vi "PathPlanner_PathFinder_GetGridPos.vi"(11 "RealGridPos":T2 {"Y" format="%14.3f"; "X" format="%14.3f"}) -> (1 "HashCode":i32, 3 "GridPosition":T1)   [LabVIEW 2019, in "PathPlanner24.lvlib"]
doc: "Internal function. Not to be used by end users."
uses:
  PathPlanner24.lvlib
  <vilib>/Rock Robotics/WPI/ThirdParty/JAS_Junk/TrajLib/TypeDef/TRANSLATION2D.ctl
  TypeDef/PathPlannerFinderGridPosition.ctl
  PathPlanner_GridPosition_Get.vi
  PathPlanner_PathFinder_Globals.vi
  <vilib>/Rock Robotics/WPI/ThirdParty/JAS_Junk/TrajLib/Trajectory_Library.lvlib
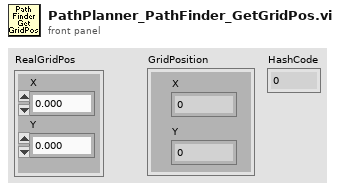
[diagram p1: front panel]
types:
  T1 = typedef "PathPlanner24.lvlib/PathPlannerFinderGridPosition.ctl" = cluster{"X":i32, "Y":i32}
  T2 = typedef "Trajectory_Library.lvlib/TRANSLATION2D.ctl" = cluster{"X":dbl, "Y":dbl}
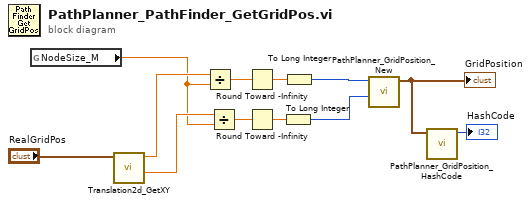
[diagram p0: block diagram]
diagram:
  n1 = global read "PathPlanner_PathFinder_Globals.vi" "NodeSize_M"() -> (w7:dbl)
  n2 = call <vilib>:"Translation2d_GetXY.vi"("In Translation"="RealGridPos") -> ("Y"=w8:dbl, "X"=w9:dbl)  [unwired: 9 in]
  n3 = Divide(x=w9, y=w7) -> (x/y=w12:dbl)
  n4 = Divide(x=w8, y=w7) -> (x/y=w11:dbl)
  n5 = Round Toward -Infinity(1:w12) -> (0:w6:dbl)
  n6 = Round Toward -Infinity(1:w11) -> (0:w5:dbl)
  n7 = To Long Integer(number=w5) -> (32bit integer=w3:i32)
  n8 = To Long Integer(number=w6) -> (32bit integer=w4:i32)
  n9 = call "PathPlanner_GridPosition_New.vi"("Int Y"=w3, "Int X"=w4) -> ("GridPosition"=w2:T1)  [unwired: 9 in]
  "GridPosition" <- w2
  n10 = call "PathPlanner_GridPosition_HashCode.vi"("GridPosition"=w2) -> ("HashCode"=→"HashCode":i32)  [unwired: 10 in]
